vi "Stop.vi"(11 "Engine":refnum<k7>) -> (0 "Error Out":errorcluster)   [LabVIEW 2021, in "Seq Edit Quick Drop.lvlib"]
uses:
  Seq Edit Quick Drop.lvlib
  Message.ctl
  Command.ctl
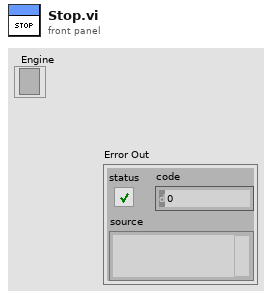
[diagram p1: front panel]
types:
  T1 = typedef "Seq Edit Quick Drop.lvlib/Message.ctl" = cluster{"cmd":T2, "data":variant}
  T2 = typedef "Seq Edit Quick Drop.lvlib/Command.ctl" = enum16{"Init", "Get Application Manager", "Shortcut Activated", "Display Tools", "Tool Selected", "Timeout", "Error", "Close"}
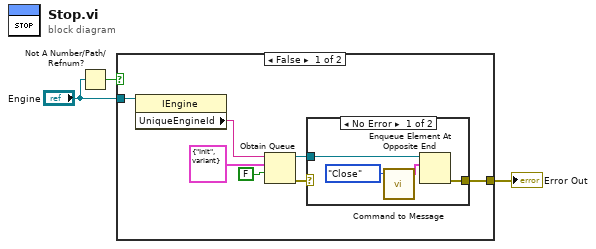
[diagram p0: block diagram]
diagram:
  n1 = Not A Number/Path/Refnum?(number/path/refnum="Engine") -> (NaN/Path/Refnum?=w2:bool)
  n2 = case shown="False" w2 {
    tunnel: "Engine" -> [w10 _]
    tunnel: [w4 _] -> w1
    frame False {
      n3 = property class="IEngine"(reference=w10) -> ("UniqueEngineId"=w9:string)  [unwired: 1 in, 2 out]
      n4 = Obtain Queue(name (unnamed)=w9, element data type=T1 {"cmd"=enum."Init", "data"=variant} ("msg"), create if not found? (T)=FALSE) -> (queue out=w6:refnum<queue>, error out=w5:errorcluster)  [unwired: 2 in, 1 out]
      n5 = case shown="No Error" w5 {
        selector: w5 -> [_ w15]
        tunnel: w6 -> [w12 _]
        tunnel: [w11 w15] -> w4
        frame No Error {
          n6 = call "Command to Message.vi"("cmd"=Command."Close") -> ("msg"=w13:T1)  [unwired: 4 in]
          n7 = Enqueue Element At Opposite End(queue=w12, element=w13) -> (error out=w11:errorcluster)  [unwired: 2 in, 2 out]
        }
        frame Error {
        }
      }
    }
    frame True {
    }
  }
  "Error Out" <- w1
